vi "XYZChangetoArrayCombination.vi"(5 "Stave Orientation":bool, 6 "N calib points":i32=8, 7 "Stave Coordinate System":enum16{"Tooling Pins", "Bus Tape"}(ring), 8 "N pics captured":i32=10, 9 "z change":dbl, 10 "y change":dbl, 11 "x change":dbl) -> (1 "Array of Coords to go to":dbl[][](array[numeric]))   [LabVIEW 2016]
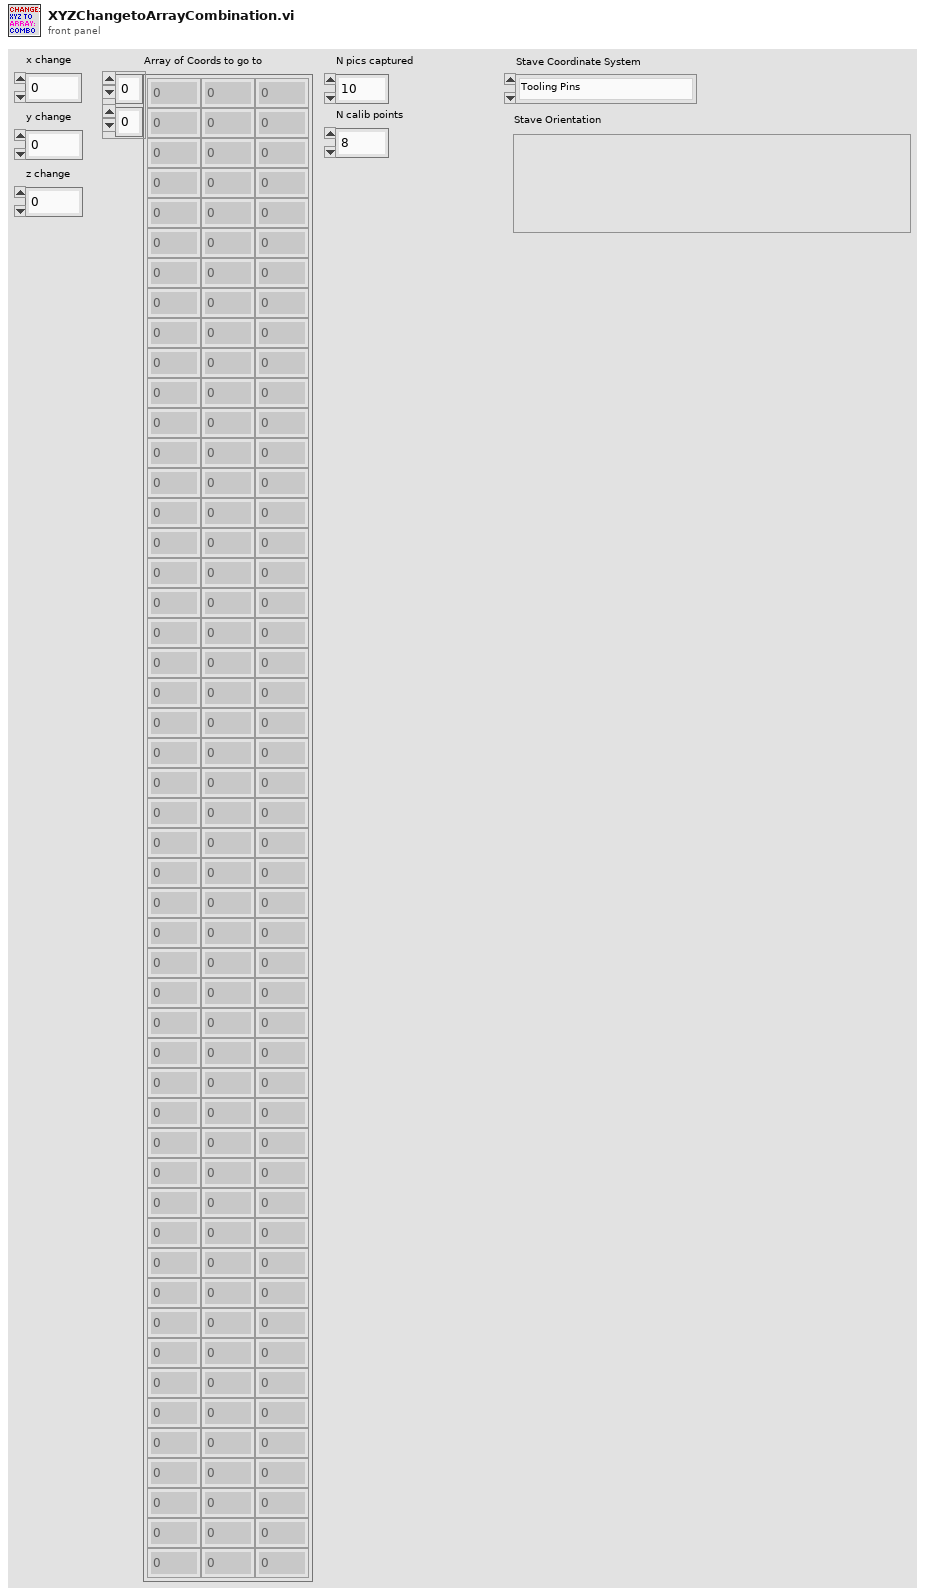
[diagram p1: front panel]
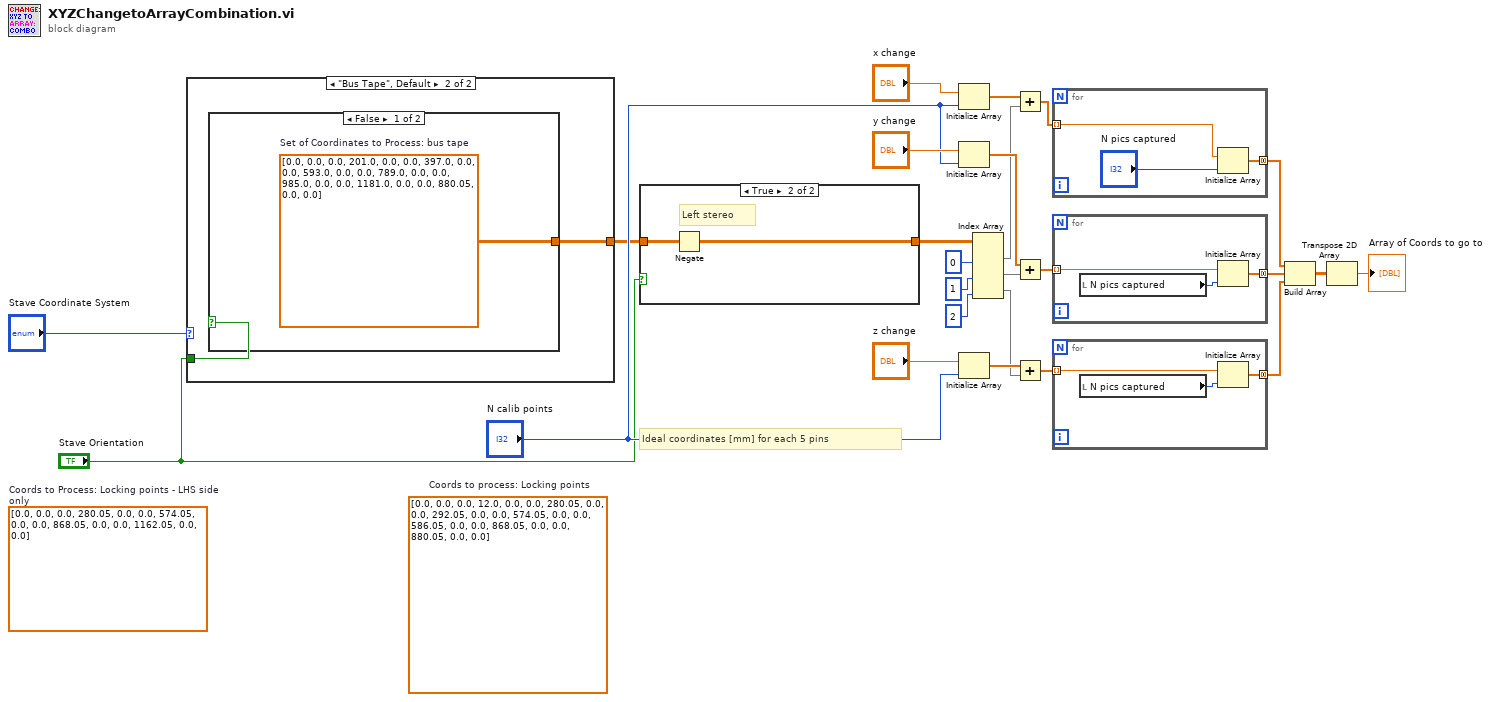
[diagram p0: block diagram]
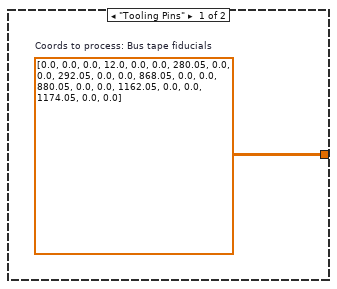
[diagram p3: hidden frame]
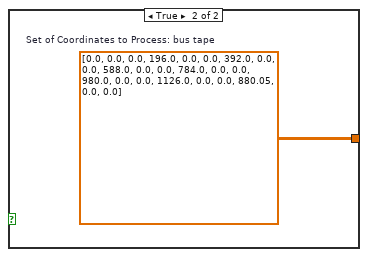
[diagram p4: hidden frame]
diagram:
  (unwired) dbl[][] [[0.0, 0.0, 0.0], [12.0, 0.0, 0.0], [280.05, 0.0, 0.0], [292.05, 0.0, 0.0], [574.05, 0.0, 0.0], [586.05, 0.0, 0.0], [868.05, 0.0, 0.0], [880.05, 0.0, 0.0]]  # Coords to process: Locking points
  (unwired) dbl[][] [[0.0, 0.0, 0.0], [280.05, 0.0, 0.0], [574.05, 0.0, 0.0], [868.05, 0.0, 0.0], [1162.05, 0.0, 0.0]]  # Coords to Process: Locking points - LHS side only
  # "Ideal coordinates [mm] for each 5 pins"
  n1 = case shown="\"Bus Tape\", Default" "Stave Coordinate System" {
    tunnel: [w26 w28] -> w3
    tunnel: "Stave Orientation" -> [_ w27]
    frame "Tooling Pins" {
      w26 = dbl[][] [[0.0, 0.0, 0.0], [12.0, 0.0, 0.0], [280.05, 0.0, 0.0], [292.05, 0.0, 0.0], [868.05, 0.0, 0.0], [880.05, 0.0, 0.0], [1162.05, 0.0, 0.0], [1174.05, 0.0, 0.0]]  # Coords to process: Bus tape fiducials
    }
    frame "Bus Tape", Default {
      n2 = case shown="False" w27 {
        tunnel: [w29 w30] -> w28
        frame False {
          w29 = dbl[][] [[0.0, 0.0, 0.0], [201.0, 0.0, 0.0], [397.0, 0.0, 0.0], [593.0, 0.0, 0.0], [789.0, 0.0, 0.0], [985.0, 0.0, 0.0], [1181.0, 0.0, 0.0], [880.05, 0.0, 0.0]]  # Set of Coordinates to Process: bus tape
        }
        frame True {
          w30 = dbl[][] [[0.0, 0.0, 0.0], [196.0, 0.0, 0.0], [392.0, 0.0, 0.0], [588.0, 0.0, 0.0], [784.0, 0.0, 0.0], [980.0, 0.0, 0.0], [1126.0, 0.0, 0.0], [880.05, 0.0, 0.0]]  # Set of Coordinates to Process: bus tape
        }
      }
    }
  }
  n3 = case shown="True" "Stave Orientation" {
    tunnel: w3 -> [w31 w33]
    tunnel: [w31 w32] -> w2
    frame False {
      # "Right stereo, Sutcliffe patterns"
    }
    frame True {
      # "Left stereo"
      n4 = Negate(x=w33) -> (-x=w32:dbl[][])
    }
  }
  n5 = Initialize Array("x change", "N calib points") -> (w20:dbl[])
  n6 = Initialize Array("y change", "N calib points") -> (w19:dbl[])
  n7 = Initialize Array("z change", "N calib points") -> (w18:dbl[])
  n8 = Index Array(array=w2, index (col) #1=0 ("disabled index (col)"), index (col) #2=1 ("index (col)"), index (col) #3=2 ("index (col)")) -> (element #1=w11:dbl[], element #2=w8:dbl[], element #3=w7:dbl[])  [unwired: 3 in]
  n9 = Add(x=w20, y=w11) -> (x+y=w12:dbl[])
  n10 = Add(x=w19, y=w8) -> (x+y=w14:dbl[])
  n11 = Add(x=w18, y=w7) -> (x+y=w13:dbl[])
  n12 = for {
    tunnel: w12 -> [w35] mode=indexing
    tunnel: [w34] -> w21 mode=concatenating
    n13 = Initialize Array(w35, "N pics captured") -> (w34:dbl[])
  }
  n14 = for {
    tunnel: w14 -> [w39] mode=indexing
    tunnel: [w38] -> w22 mode=concatenating
    n15 = local read "N pics captured"() -> (w37:i32)
    n16 = Initialize Array(w39, w37) -> (w38:dbl[])
  }
  n17 = for {
    tunnel: w13 -> [w42] mode=indexing
    tunnel: [w41] -> w23 mode=concatenating
    n18 = local read "N pics captured"() -> (w40:i32)
    n19 = Initialize Array(w42, w40) -> (w41:dbl[])
  }
  n20 = Build Array(w21, w22, w23) -> (w24:dbl[][])
  n21 = Transpose 2D Array(2D array=w24) -> (transposed array=→"Array of Coords to go to":dbl[][])
